vi "Compare_Calib_Files.vi"(3 "Instrument type":T1=enum."Cross wire velocity", 4 "Calib file Orig":path=path "/iMac_3 HD/Users/Hong(6%)/calib/XW Ch 1 7_10_02_5", 5 "Calib file New":path=path "/iMac_3 HD/Users/Hong(6%)/calib/XW Ch 1 7_10_02_6") -> (0 "Calib Time Separation (Hours)":dbl format="%.2f", 1 "% Change":dbl format="%.2f", 2 "Calib name":string)   [LabVIEW 2010]
uses:
  Controls/Cal_Inst_type.ctl
  Controls/Inst_type.ctl
panel:
  out "U1 % Change":dbl format="%.4f"
  out "U2 % Change":dbl format="%.4f"
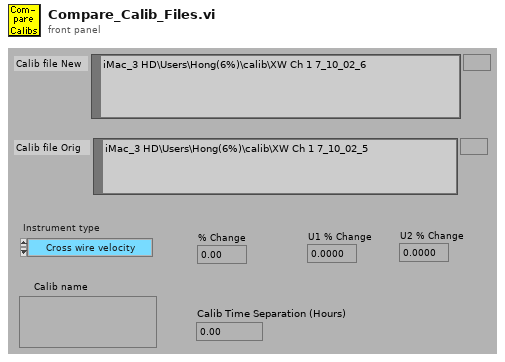
[diagram p1: front panel]
types:
  T1 = typedef "Cal_Inst_type.ctl" = enum16{"Propeller anemometer", "Pressure Transducer", "Hot wire", "Cross wire velocity", "Cross wire angle", "Generic Linear", "Generic Polynomial", "Generic BackPoly", "Fast FID", "Thermocouple", "Cold wire", "Pulsed Wire"}
  T2 = typedef "Inst_type.ctl" = enum16{"Propeller anemometer", "Raw voltage", "Pressure Transducer", "Pitot-static tube", "Preston tube", "Hot wire", "Cross wire 1", "Cross wire 2", "Generic Linear", "Generic Polynomial", "Generic BackPoly", "Fast FID", "Thermocouple", "Cold wire", "Pulsed Wire", "LDA Vel", "LDA Tran time", "LDA Arr time"}
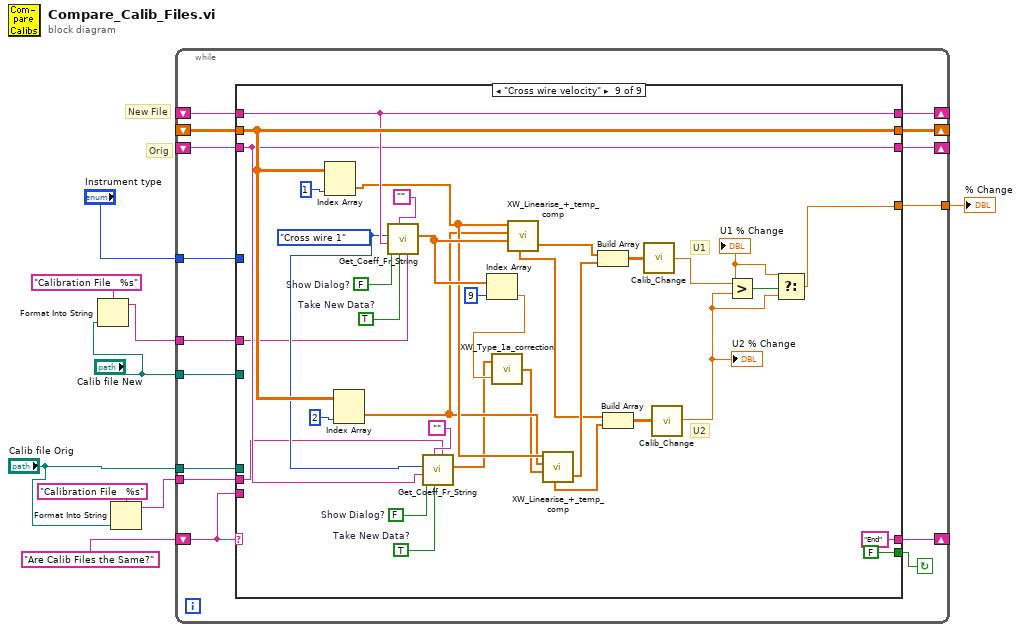
[diagram p0: block diagram]
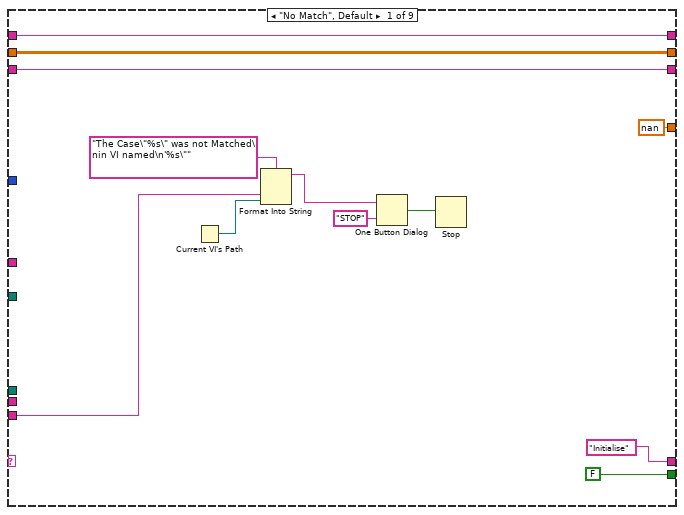
[diagram p2: hidden frame]
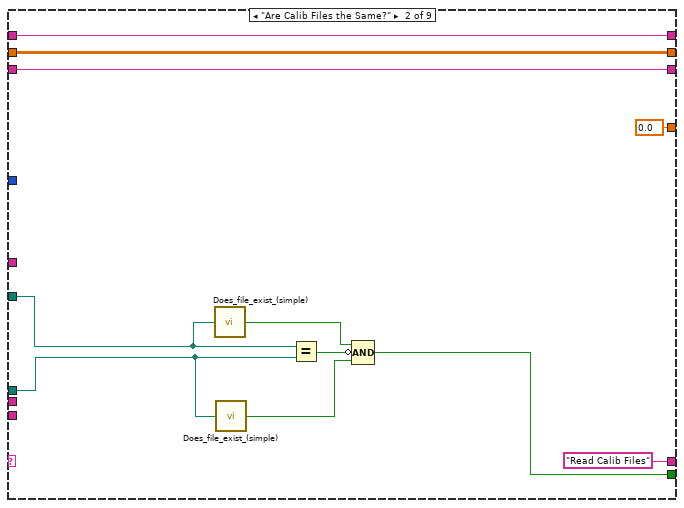
[diagram p3: hidden frame]
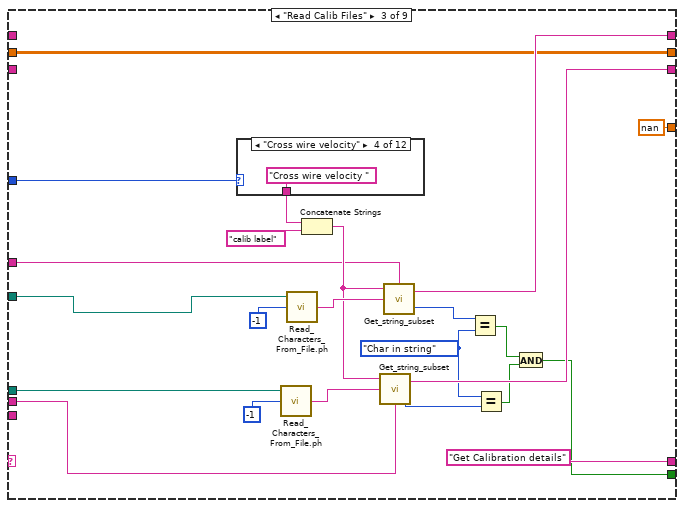
[diagram p4: hidden frame]
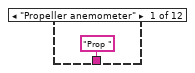
[diagram p5: hidden frame]
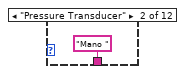
[diagram p6: hidden frame]
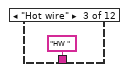
[diagram p7: hidden frame]
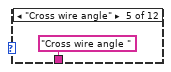
[diagram p8: hidden frame]
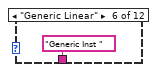
[diagram p9: hidden frame]
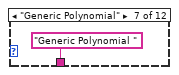
[diagram p10: hidden frame]
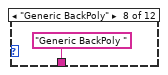
[diagram p11: hidden frame]
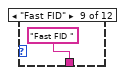
[diagram p12: hidden frame]
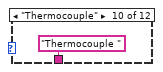
[diagram p13: hidden frame]
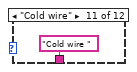
[diagram p14: hidden frame]
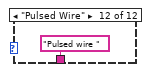
[diagram p15: hidden frame]
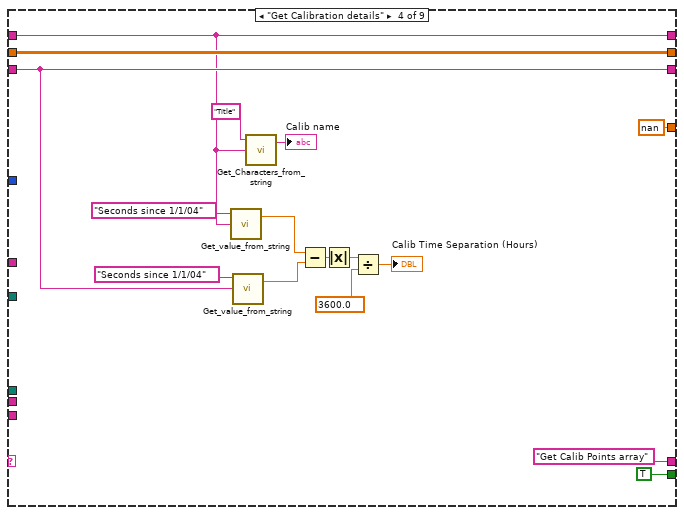
[diagram p16: hidden frame]
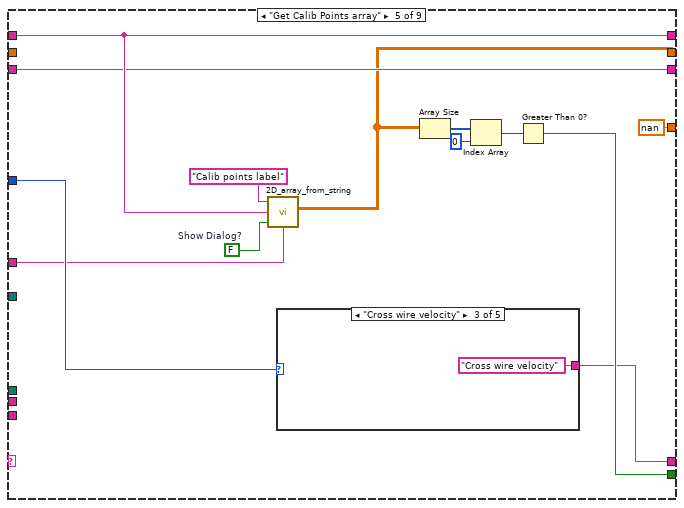
[diagram p17: hidden frame]
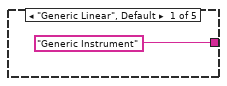
[diagram p18: hidden frame]
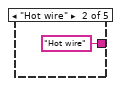
[diagram p19: hidden frame]
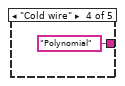
[diagram p20: hidden frame]
diagram:
  # "New File"
  # "Orig"
  n1 = Format Into String(format string="Calibration File   %s", "Calib file New") -> (resulting string=w2:string)  [unwired: 2 in, 1 out]
  n2 = Format Into String(format string="Calibration File   %s", "Calib file Orig") -> (resulting string=w1:string)  [unwired: 2 in, 1 out]
  n3 = while {
    tunnel: "Calib file Orig" -> [w12]
    tunnel: "Calib file New" -> [w13]
    tunnel: [w14] -> w7
    shift-left: _ -> [w15]
    shift-right: [w16] -> _
    shift-left: _ -> [w17]
    shift-right: [w19] -> _
    tunnel: "Instrument type" -> [w21]
    shift-left: _ -> [w18]
    shift-right: [w20] -> _
    shift-left: "Are Calib Files the Same?" -> [w22]
    shift-right: [w23] -> _
    tunnel: w2 -> [w11]
    tunnel: w1 -> [w10]
    stop <- w24 continue-if-true
    n4 = case shown="\"Cross wire velocity\"" w22 {
      tunnel: [FALSE w39 w53 TRUE w102 FALSE FALSE FALSE FALSE] -> w24
      tunnel: ["Initialise" "Read Calib Files" "Get Calibration details" "Get Calib Points array" w100 "End" "End" "End" "End"] -> w23
      tunnel: w22 -> [w31 _ _ _ _ _ _ _ _]
      tunnel: w21 -> [_ _ w65 _ w107 _ _ _ _]
      tunnel: [w28 w47 w64 w84 w109 w135 w144 w172 w228] -> w20
      tunnel: [w27 w45 w61 w95 w108 w128 w143 w171 w222] -> w19
      tunnel: w18 -> [w28 w47 _ w84 w109 w135 w144 w172 w228]
      tunnel: w17 -> [w27 w45 _ w95 w108 w128 w143 w171 w222]
      tunnel: [w26 w46 w60 w98 w106 w142 w152 w185 w238] -> w16
      tunnel: w15 -> [w26 w46 w60 w98 _ w142 w152 w185 w238]
      tunnel: [nan ("% Change") 0.0 ("% Change") nan ("% Change") nan ("% Change") nan ("% Change") w140 w147 w180 w234] -> w14
      tunnel: w13 -> [_ w38 w50 _ _ _ _ _ _]
      tunnel: w12 -> [_ w37 w51 _ _ _ _ _ _]
      tunnel: w11 -> [_ _ w49 _ w99 w118 _ _ w209]
      tunnel: w10 -> [_ _ w48 _ _ w117 _ _ w208]
      frame "No Match", Default {
        n5 = Current VI's Path() -> (path=w30:path)
        n6 = Format Into String(format string="The Case\"%s\" was not Matched\nin VI named\n'%s\"" ("Format String"), w31, w30) -> (resulting string=w34:string)  [unwired: 2 in, 1 out]
        n7 = One Button Dialog(message=w34, button name ("OK")="STOP") -> (true=w32:bool)
        n8 = Stop(stop? (T)=w32) -> ()
      }
      frame "Are Calib Files the Same?" {
        n9 = call "Does_file_exist_(simple).vi"("Pathname"=w38) -> ("exists?"=w42:bool)
        n10 = call "Does_file_exist_(simple).vi"("Pathname"=w37) -> ("exists?"=w40:bool)
        n11 = Equal?(x=w38, y=w37) -> (x = y?=w41:bool)
        n12 = Compound Arithmetic op=AND(w42, invert w41, w40) -> (w39:bool)
      }
      frame "Read Calib Files" {
        w57 = enum16{"Char in string", "Char not in string"}."Char in string" ("Status")
        n13 = case shown="\"Cross wire velocity\"" w65 {
          tunnel: ["Prop " "Mano " "HW " "Cross wire velocity " "Cross wire angle " "Generic Inst " "Generic Polynomial " "Generic BackPoly " "Fast FID " "Thermocouple " "Cold wire " "Pulsed wire "] -> w66
          frame "Propeller anemometer" {
          }
          frame "Pressure Transducer" {
          }
          frame "Hot wire" {
          }
          frame "Cross wire velocity" {
          }
          frame "Cross wire angle" {
          }
          frame "Generic Linear" {
          }
          frame "Generic Polynomial" {
          }
          frame "Generic BackPoly" {
          }
          frame "Fast FID" {
          }
          frame "Thermocouple" {
          }
          frame "Cold wire" {
          }
          frame "Pulsed Wire" {
          }
        }
        n14 = call "Read_Characters_From_File.ph.vi"("file path (dialog if empty)"=w51, "number of characters (all:-1)"=-1) -> ("character string"=w63:string)  [unwired: 7 out]
        n15 = call "Read_Characters_From_File.ph.vi"("file path (dialog if empty)"=w50, "number of characters (all:-1)"=-1) -> ("character string"=w68:string)  [unwired: 7 out]
        n16 = Concatenate Strings(w66, "calib label") -> (w59:string)
        n17 = call "Get_string_subset.vi"("String Name"=w48, "String to split"=w63, "File Label"=w59) -> ("Status"=w56:enum16{"Char in string", "Char not in string"}, "Output string"=w61:string)  [unwired: 1 in]
        n18 = call "Get_string_subset.vi"("String Name"=w49, "String to split"=w68, "File Label"=w59) -> ("Status"=w58:enum16{"Char in string", "Char not in string"}, "Output string"=w64:string)  [unwired: 1 in]
        n19 = Equal?(x=w58, y=w57) -> (x = y?=w54:bool)
        n20 = Equal?(x=w57, y=w56) -> (x = y?=w55:bool)
        n21 = And(x=w54, y=w55) -> (x .and. y?=w53:bool)
      }
      frame "Get Calibration details" {
        n22 = call "Get_value_from_string.vi"("Input string"=w84, "Variable name"="Seconds since 1/1/04") -> ("Value"=w94:dbl)  [unwired: 1 in, 1 out]
        n23 = call "Get_value_from_string.vi"("Input string"=w95, "Variable name"="Seconds since 1/1/04") -> ("Value"=w93:dbl)  [unwired: 1 in, 1 out]
        n24 = call "Get_Characters_from_string.vi"("Input string"=w84, "Variable name"="Title") -> ("Value"=→"Calib name":string)  [unwired: 1 in, 1 out]
        n25 = Subtract(x=w94, y=w93) -> (x-y=w92:dbl)
        n26 = Absolute Value(x=w92) -> (abs(x)=w83:dbl)
        n27 = Divide(x=w83, y=3600.0) -> (x/y=→"Calib Time Separation (Hours)":dbl)
      }
      frame "Get Calib Points array" {
        w111 = FALSE  # Show Dialog?
        n28 = call "2D_array_from_string.vi"("String Name"=w99, "Show Dialog?"=w111, "Input string"=w109, "Array title"="Calib points label") -> ("2D data array"=w106:dbl[][])
        n29 = case shown="\"Cross wire velocity\"" w107 {
          tunnel: ["Generic Instrument" "Hot wire" "Cross wire velocity" "Polynomial" "Polynomial"] -> w100
          frame "Generic Linear", Default {
          }
          frame "Hot wire" {
          }
          frame "Cross wire velocity" {
          }
          frame "Cold wire" {
          }
          frame "Fast FID" {
          }
        }
        n30 = Array Size(array=w106) -> (size(s)=w105:i32[])
        n31 = Index Array(array=w105, index=0 ("Index")) -> (element=w103:i32)
        n32 = Greater Than 0?(x=w103) -> (x > 0?=w102:bool)
      }
      frame "Hot wire" {
        w132 = TRUE  # Take New Data?
        w131 = FALSE  # Show Dialog?
        w133 = TRUE  # Take New Data?
        w134 = FALSE  # Show Dialog?
        # "New Calib"
        # "Original calib corrected to new calib temperture"
        n33 = call "Get_Coeff_Fr_String.vi"("String Name"=w118, "Take New Data?"=w133, "Prefix"="", "Show Dialog?"=w134, "Sub String"=w135, "Inst type"=Inst_type."Hot wire") -> ("Calib Constants"=w125:dbl[])  [unwired: 3 in, 1 out]
        n34 = call "Get_Coeff_Fr_String.vi"("String Name"=w117, "Take New Data?"=w132, "Prefix"="", "Show Dialog?"=w131, "Sub String"=w128, "Inst type"=Inst_type."Hot wire") -> ("Calib Constants"=w121:dbl[])  [unwired: 3 in, 1 out]
        n35 = Index Array(array=w125, index=3) -> (element=w120:dbl)
        n36 = Index Array(array=w142, index (col)=1 ("Index")) -> (element=w127:dbl[])  [unwired: 1 in]
        n37 = call "HW_Linearise_+_temp_comp.vi"("Caib const"=w125, "HW voltage"=w127) -> ("Velocity"=w124:dbl[])  [unwired: 3 in, 1 out]
        n38 = call "SW_Type_1a_correction.vi"("Tmeas (degC)"=w120, "Calib consts."=w121) -> ("Corrected calib consts."=w119:dbl[])
        n39 = call "HW_Linearise_+_temp_comp.vi"("Caib const"=w119, "HW voltage"=w127) -> ("Velocity"=w123:dbl[])  [unwired: 3 in, 1 out]
        n40 = Build Array(w124, w123) -> (w122:dbl[][])
        n41 = call "Calib_Change.vi"("Eng Units"=w122) -> ("% Change"=w140:dbl)
      }
      frame "Generic Instrument" {
        n42 = Index Array(array=w152, index (col)=1 ("Index")) -> (element=w149:dbl[])  [unwired: 1 in]
        n43 = for {
          N: 2 -> [_]
          tunnel: w143 -> [w162]
          tunnel: w144 -> [w158]
          tunnel: w149 -> [w155]
          tunnel: [w153] -> w148 mode=indexing
          i -> [w163]
          w159 = FALSE  # Show Dialog?
          n44 = case shown="1" w163 {
            tunnel: w162 -> [_ w170]
            tunnel: [w169 w170] -> w161
            tunnel: w158 -> [w169 _]
            frame 0, Default {
            }
            frame 1 {
            }
          }
          n45 = call "Get_value_from_string.vi"("Show Dialog?"=w159, "Input string"=w161, "Variable name"="Coeff A") -> ("Value"=w160:dbl)  [unwired: 1 out]
          n46 = call "Get_value_from_string.vi"("Show Dialog?"=w159, "Input string"=w161, "Variable name"="Coeff B") -> ("Value"=w154:dbl)  [unwired: 1 out]
          n47 = for {
            tunnel: w160 -> [w167]
            tunnel: w155 -> [w166] mode=indexing
            tunnel: w154 -> [w165]
            tunnel: [w164] -> w153 mode=indexing
            n48 = Subtract(x=w166, y=w167) -> (x-y=w168:dbl)
            n49 = Divide(x=w168, y=w165) -> (x/y=w164:dbl)
          }
        }
        n50 = call "Calib_Change.vi"("Eng Units"=w148) -> ("% Change"=w147:dbl)
      }
      frame "Polynomial" {
        n51 = Index Array(array=w185, index (col)=1 ("Index")) -> (element=w182:dbl[])  [unwired: 1 in]
        n52 = Build Array("Coeff A", "Coeff B", "Coeff C", "Coeff D") -> (w175:string[])
        n53 = for {
          N: 2 -> [_]
          tunnel: w171 -> [w193]
          tunnel: w172 -> [w192]
          tunnel: w182 -> [w191]
          tunnel: [w190] -> w181 mode=indexing
          tunnel: w175 -> [w187]
          i -> [w194]
          w189 = FALSE  # Show Dialog?
          n54 = case shown="1" w194 {
            tunnel: w193 -> [_ w207]
            tunnel: [w206 w207] -> w188
            tunnel: w192 -> [w206 _]
            frame 0, Default {
            }
            frame 1 {
            }
          }
          n55 = for {
            tunnel: w189 -> [w199]
            tunnel: w188 -> [w198]
            tunnel: w187 -> [w197] mode=indexing
            tunnel: [w195] -> w186 mode=indexing
            n56 = call "Get_value_from_string.vi"("Show Dialog?"=w199, "Input string"=w198, "Variable name"=w197) -> ("Status"=w200:enum16{"Char in string", "Char not in string"}, "Value"=w196:dbl)
            n57 = case shown="\"Char not in string\"" w200 {
              tunnel: w196 -> [w201 _]
              tunnel: [w201 0.0 ("Value")] -> w195
              frame "Char in string" {
              }
              frame "Char not in string" {
              }
            }
          }
          n58 = for {
            tunnel: w191 -> [w205] mode=indexing
            tunnel: [w204] -> w190 mode=indexing
            tunnel: w186 -> [w203]
            n59 = call "Polynomial_convert.vi"("Calib constants"=w203, "Voltage"=w205) -> ("Eng Values"=w204:dbl)  [unwired: 4 out]
          }
        }
        n60 = call "Calib_Change.vi"("Eng Units"=w181) -> ("% Change"=w180:dbl)
      }
      frame "Cross wire velocity" {
        w225 = TRUE  # Take New Data?
        w224 = FALSE  # Show Dialog?
        w229 = TRUE  # Take New Data?
        w230 = FALSE  # Show Dialog?
        w213 = Inst_type."Cross wire 1" ("Inst type")
        # "U2"
        # "U1"
        n61 = Index Array(array=w238, index (col)=1 ("Index")) -> (element=w221:dbl[])  [unwired: 1 in]
        n62 = Index Array(array=w238, index (col)=2 ("Index")) -> (element=w220:dbl[])  [unwired: 1 in]
        n63 = call "Get_Coeff_Fr_String.vi"("String Name"=w209, "Take New Data?"=w229, "Prefix"="", "Show Dialog?"=w230, "Sub String"=w228, "Inst type"=w213) -> ("Calib Constants"=w226:dbl[])  [unwired: 3 in, 1 out]
        n64 = call "Get_Coeff_Fr_String.vi"("String Name"=w208, "Take New Data?"=w225, "Prefix"="", "Show Dialog?"=w224, "Sub String"=w222, "Inst type"=w213) -> ("Calib Constants"=w211:dbl[])  [unwired: 3 in, 1 out]
        n65 = Index Array(array=w226, index=9) -> (element=w212:dbl)
        n66 = call "XW_Type_1a_correction.vi"("Tmeas (degC)"=w212, "Calib consts."=w211) -> ("Corrected calib consts."=w210:dbl[])
        n67 = call "XW_Linearise_+_temp_comp.vi"("Calib const"=w226, "XW2 voltage"=w220, "XW1 voltage"=w221) -> ("U1"=w216:dbl[], "U2"=w215:dbl[])  [unwired: 1 in, 2 out]
        n68 = call "XW_Linearise_+_temp_comp.vi"("Calib const"=w210, "XW2 voltage"=w220, "XW1 voltage"=w221) -> ("U1"=w219:dbl[], "U2"=w217:dbl[])  [unwired: 1 in, 2 out]
        n69 = Build Array(w216, w219) -> (w218:dbl[][])
        n70 = Build Array(w215, w217) -> (w214:dbl[][])
        n71 = call "Calib_Change.vi"("Eng Units"=w218) -> ("% Change"=w236:dbl)
        "U1 % Change" <- w236
        n72 = call "Calib_Change.vi"("Eng Units"=w214) -> ("% Change"=w235:dbl)
        "U2 % Change" <- w235
        n73 = Greater?(x=w236, y=w235) -> (0:w237:bool)
        n74 = Select(t=w236, s=w237, f=w235) -> (s? t:f=w234:dbl)
      }
    }
  }
  "% Change" <- w7
